vi "GetDims.vi"() -> ()   [LabVIEW 2020]
panel:
  out "dims":cluster{"name":string, "size":u64}[](array[cluster])
  out "vars":T1(array[cluster])
  in  "FilePath":path
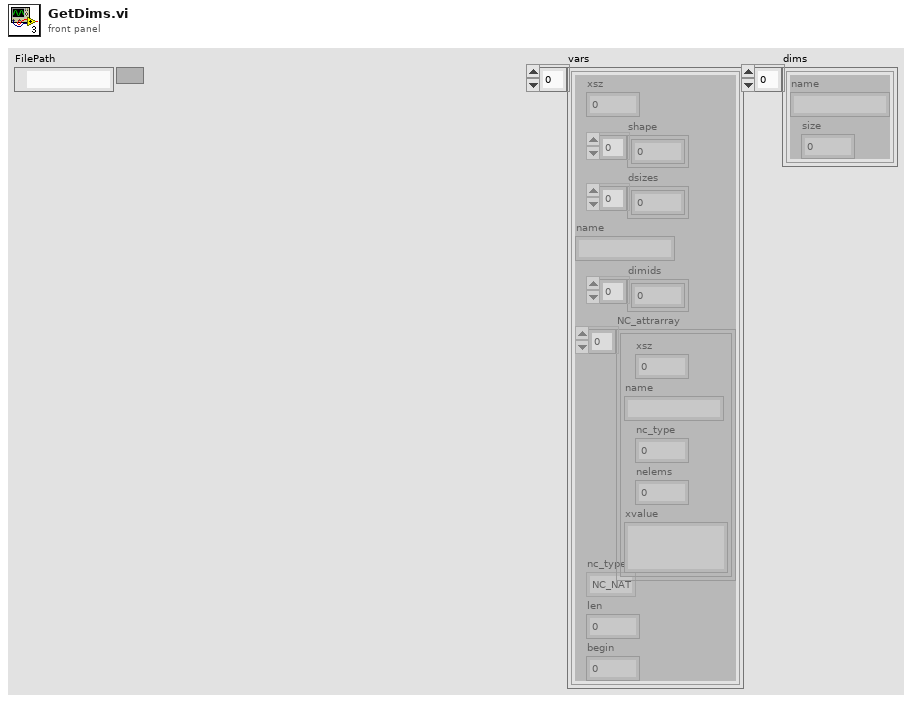
[diagram p1: front panel]
types:
  T1 = cluster{"xsz":u64, "shape":u64[], "dsizes":u64[], "name":string, "dimids":u64[], "NC_attrarray":cluster{"xsz":u64, "name":string, "nc_type":u16, "nelems":u64, "xvalue":string}[], "nc_type":enum16{"NC_NAT", "NC_BYTE", "NC_CHAR", "NC_SHORT", "NC_INT", "NC_FLOAT", "NC_DOUBLE"}, "len":u64, "begin":u64}[]
  T2 = cluster{"numrecs":u64, "dims":cluster{"name":string, "size":u64}[], "attrs":cluster{"xsz":u64, "name":string, "nc_type":u16, "nelems":u64, "xvalue":string}[], "vars":cluster{"xsz":u64, "shape":u64[], "dsizes":u64[], "name":string, "dimids":u64[], "NC_attrarray":cluster{"xsz":u64, "name":string, "nc_type":u16, "nelems":u64, "xvalue":string}[], "nc_type":enum16{"NC_NAT", "NC_BYTE", "NC_CHAR", "NC_SHORT", "NC_INT", "NC_FLOAT", "NC_DOUBLE"}, "len":u64, "begin":u64}[]}
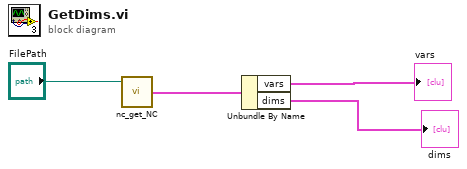
[diagram p0: block diagram]
diagram:
  n1 = call "nc_get_NC.vi"("FilePath"="FilePath") -> ("NC"=w3:T2)  [unwired: 1 in, 3 out]
  n2 = Unbundle By Name(w3) -> ("vars"=→"vars":T1, "dims"=→"dims":cluster{"name":string, "size":u64}[])
